vi "XNET UDP Socket Read.vi"   [LabVIEW 2018]
doc: "Reads a datagram from a UDP socket."
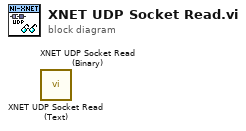
[diagram p0: block diagram]
diagram:
  n1 = call "XNET UDP Socket Read (Text).vi"() -> ()  [unwired: 7 in, 5 out]
  n2 = call "XNET UDP Socket Read (Binary).vi"() -> ()  [unwired: 7 in, 5 out]
